vi "MGI Center Callee in Caller.vi"(8 "Error In":errorcluster, 10 "Callee VI Refnum (Caller)":refnum<vi>, 11 "Caller VI Refnum (Callee's Caller)":refnum<vi>) -> (0 "Error Out":errorcluster)   [LabVIEW 2016]
doc: "This VI is designed to center a callee VI's window in a caller VI's window.\n\nAuthored by Brandon Steele\nsupport@mooregoodideas.com\nwww.mooregoodideas.com\n\nCopyright (c) 2010, Moore Good Ideas, Inc.\n\nAll rights reserved.\n\nRedistribution and use in source and binary forms, with or without modification, are permitted provided that the following conditions are met:\n\n * Redistributions of source code must retain the above copyright notice, this list of conditions and the following disclaimer.\n * Redistributions in binary form must reproduce the above copyright notice, this list of conditions and the following disclaimer in the documentation and/or other materials provided with the distribution.\n * Neither the name of Moore Good Ideas, Inc. nor the names of its contributors may be used to endorse or promote products derived from this software without specific prior written permission.\n\nTHIS SOFTWARE IS PROVIDED BY THE COPYRIGHT HOLDERS AND CONTRIBUTORS \"AS IS\" AND ANY EXPRESS OR IMPLIED WARRANTIES, INCLUDING, BUT NOT LIMITED TO, THE IMPLIED WARRANTIES OF MERCHANTABILITY AND FITNESS FOR A PARTICULAR PURPOSE ARE DISCLAIMED. IN NO EVENT SHALL THE COPYRIGHT OWNER OR CONTRIBUTORS BE LIABLE FOR ANY DIRECT, INDIRECT, INCIDENTAL, SPECIAL, EXEMPLARY, OR CONSEQUENTIAL DAMAGES (INCLUDING, BUT NOT LIMITED TO, PROCUREMENT OF SUBSTITUTE GOODS OR SERVICES; LOSS OF USE, DATA, OR PROFITS; OR BUSINESS INTERRUPTION) HOWEVER CAUSED AND ON ANY THEORY OF LIABILITY, WHETHER IN CONTRACT, STRICT LIABILITY, OR TORT (INCLUDING NEGLIGENCE OR OTHERWISE) ARISING IN ANY WAY OUT OF THE USE OF THIS SOFTWARE, EVEN IF ADVISED OF THE POSSIBILITY OF SUCH DAMAGE."
uses:
  <userlib>/_MGI/Application Control/MGI VI Reference/MGI Caller's VI Reference.vi
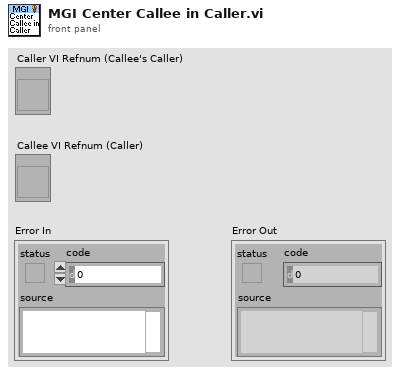
[diagram p1: front panel]
types:
  T1 = typedef "LVRectTypeDef.ctl" = cluster{"Left":i16, "Top":i16, "Right":i16, "Bottom":i16}
  T2 = cluster{"Left":i16, "Top":i16, "Right":i16, "Bottom":i16}
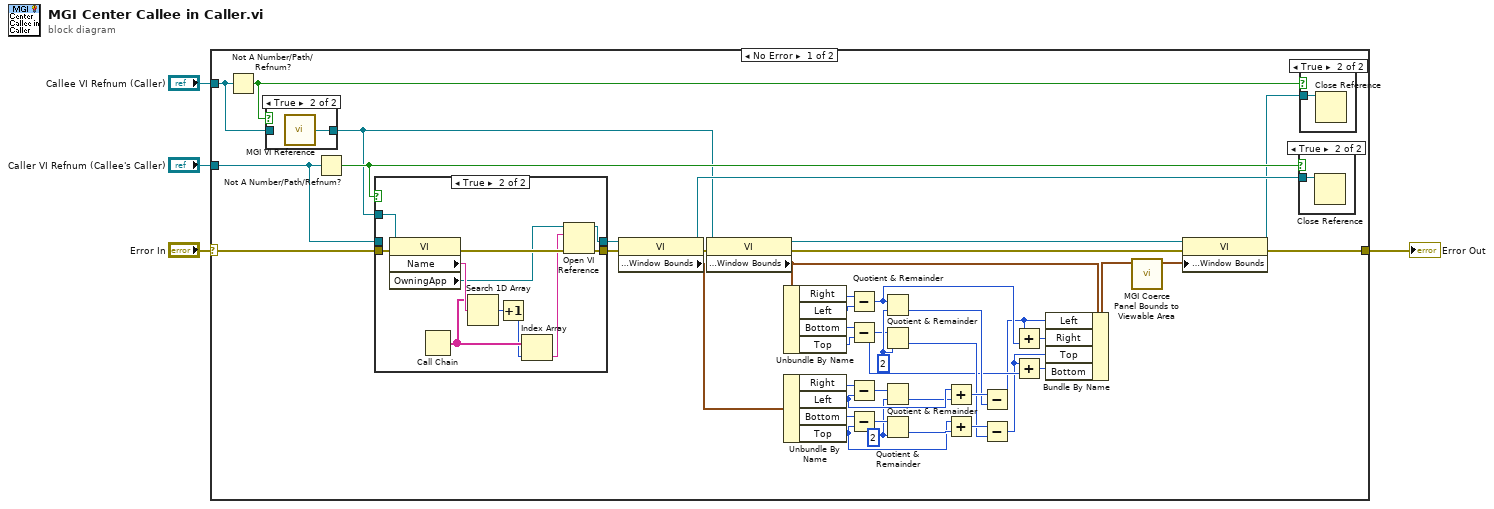
[diagram p0: block diagram]
diagram:
  n1 = case shown="No Error" "Error In" {
    selector: "Error In" -> [w21 w64]
    tunnel: [w46 w64] -> w4
    tunnel: "Caller VI Refnum (Callee's Caller)" -> [w16 _]
    tunnel: "Callee VI Refnum (Caller)" -> [w17 _]
    frame No Error {
      w39 = i16 2 ("y")
      w22 = i16 2 ("y")
      n2 = Not A Number/Path/Refnum?(number/path/refnum=w17) -> (NaN/Path/Refnum?=w18:bool)
      n3 = case shown="True" w18 {
        tunnel: w17 -> [w62 _]
        tunnel: [w62 w63] -> w12
        frame False {
        }
        frame True {
          n4 = call-poly <userlib>:"MGI VI Reference.vi"() -> ("Caller's VI Reference"=w63:refnum<vi>)  [unwired: 1 in]
        }
      }
      n5 = Not A Number/Path/Refnum?(number/path/refnum=w16) -> (NaN/Path/Refnum?=w19:bool)
      n6 = case shown="True" w19 {
        tunnel: w16 -> [w50 _]
        tunnel: [w50 w56] -> w15
        tunnel: w12 -> [_ w61]
        tunnel: w21 -> [w49 w60]
        tunnel: [w49 w57] -> w20
        frame False {
        }
        frame True {
          n7 = property class="VI"(reference=w61, error in=w60) -> (error out=w58:errorcluster, "Name"=w59:string, "OwningApp"=w53:refnum<vi>)  [unwired: 1 out]
          n8 = Call Chain() -> (call chain=w55:string[])
          n9 = Search 1D Array(1D array=w55, element=w59) -> (index of element=w52:i32)  [unwired: 1 in]
          n10 = Increment(x=w52) -> (x+1=w51:i32)
          n11 = Index Array(array=w55, index=w51) -> (element=w54:string)
          n12 = Open VI Reference(application reference (local)=w53, vi path=w54, error in (no error)=w58) -> (vi reference=w56:refnum<vi>, error out=w57:errorcluster)  [unwired: 3 in]
        }
      }
      n13 = property class="VI"(reference=w15, error in=w20) -> (reference out=w14:refnum<vi>, error out=w40:errorcluster, "Front Panel Window:Window Bounds"=w45:T1)
      n14 = property class="VI"(reference=w12, error in=w40) -> (reference out=w26:refnum<vi>, error out=w25:errorcluster, "Front Panel Window:Window Bounds"=w7:T1)
      n15 = Unbundle By Name(w7) -> ("Right"=w35:i16, "Left"=w36:i16, "Bottom"=w37:i16, "Top"=w38:i16)
      n16 = Unbundle By Name(w45) -> ("Right"=w44:i16, "Left"=w34:i16, "Bottom"=w43:i16, "Top"=w31:i16)
      n17 = Subtract(x=w35, y=w36) -> (x-y=w24:i16)
      n18 = Subtract(x=w37, y=w38) -> (x-y=w23:i16)
      n19 = Subtract(x=w44, y=w34) -> (x-y=w42:i16)
      n20 = Subtract(x=w43, y=w31) -> (x-y=w41:i16)
      n21 = Quotient & Remainder(x=w24, y=w39) -> (floor(x/y)=w29:i16)  [unwired: 1 out]
      n22 = Quotient & Remainder(x=w23, y=w39) -> (floor(x/y)=w27:i16)  [unwired: 1 out]
      n23 = Quotient & Remainder(x=w42, y=w22) -> (floor(x/y)=w33:i16)  [unwired: 1 out]
      n24 = Quotient & Remainder(x=w41, y=w22) -> (floor(x/y)=w32:i16)  [unwired: 1 out]
      n25 = Add(x=w34, y=w33) -> (x+y=w30:i16)
      n26 = Add(x=w31, y=w32) -> (x+y=w28:i16)
      n27 = Subtract(x=w30, y=w29) -> (x-y=w10:i16)
      n28 = Subtract(x=w28, y=w27) -> (x-y=w9:i16)
      n29 = Add(x=w10, y=w24) -> (x+y=w8:i16)
      n30 = Add(x=w9, y=w23) -> (x+y=w11:i16)
      n31 = Bundle By Name(cluster=w7, "Left"=w10, "Right"=w8, "Top"=w9, "Bottom"=w11) -> (w6:T1)
      n32 = call <userlib>:"MGI Coerce Panel Bounds to Viewable Area.vi"("Panel Bounds In"=w6) -> ("Panel Bounds Out"=w5:T2)  [unwired: 9 in, 1 out]
      n33 = property class="VI"(reference=w26, error in=w25, "Front Panel Window:Window Bounds"=w5) -> (reference out=w13:refnum<vi>, error out=w46:errorcluster)
      n34 = case shown="True" w19 {
        tunnel: w14 -> [_ w48]
        frame False {
        }
        frame True {
          n35 = Close Reference(reference=w48) -> ()  [unwired: 1 in, 1 out]
        }
      }
      n36 = case shown="True" w18 {
        tunnel: w13 -> [_ w47]
        frame False {
        }
        frame True {
          n37 = Close Reference(reference=w47) -> ()  [unwired: 1 in, 1 out]
        }
      }
    }
    frame Error {
    }
  }
  "Error Out" <- w4
